vi "Send.vi"(8 "error in":errorcluster, 11 "Block Upload Transfer in":refnum<class "Block Upload Sub-Block Transfer.lvclass">) -> (0 "error out":errorcluster, 3 "Block Upload Transfer out":refnum<class "Block Upload Sub-Block Transfer.lvclass">)   [LabVIEW 2020, in "CANopen.lvlib" / "SDO Manager.lvlib" / "Block Upload Sub-Block Transfer.lvclass"]
doc: "SDO block upload initiate (phase II)"
uses:
  Block Upload Sub-Block Transfer.lvclass
  D:/git/CANopen-LabVIEW/source/SDO/SDO Manager/SDO Transfer/SDO Transfer.lvclass
  SDO Transfer/SDO Transfer.lvclass/SDO Transfer.ctl
  CANopen Message/CANopen Message.lvclass/CANopen Message.ctl
  HAL/Source/Interfaces/ICommunicate/ICommunicate.lvclass
  CANopen Message/CANopen Message.lvclass
  Typedefs/Function Code.ctl
  CANopen.lvlib
  SDO Transfer/SDO Transfer.lvclass
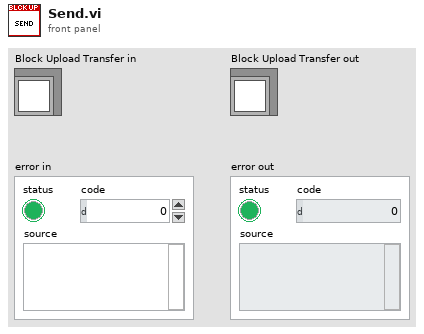
[diagram p1: front panel]
types:
  T1 = typedef "CANopen.lvlib/Function Code.ctl" = u8
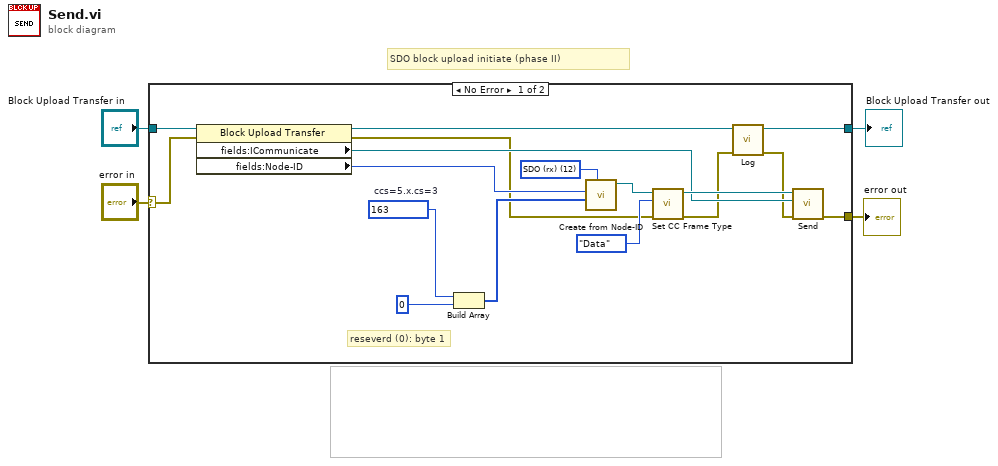
[diagram p0: block diagram]
diagram:
  # "SDO block upload initiate (phase II)"
  n1 = case shown="No Error" "error in" {
    selector: "error in" -> [w21 w22]
    tunnel: "Block Upload Transfer in" -> [w20 w23]
    tunnel: [w10 w23] -> w3
    tunnel: [w9 w22] -> w2
    frame No Error {
      w16 = T1 12 items=["NMT"=0, "EMCY/SYNC"=1, "TIME"=2, "PDO1 (tx)"=3, "PDO1 (rx)"=4, "PDO2 (tx)"=5, "PDO2 (rx)"=6, "PDO3 (tx)"=7, "PDO3 (rx)"=8, "PDO4 (tx)"=9, "PDO4 (rx)"=10, "SDO (tx)"=11, "SDO (rx)"=12, "NMT error control"=14] ("Function Code")
      w18 = u8 163  # ccs=5.x.cs=3
      # "reseverd (0): byte 1"
      n2 = property class="Block Upload Transfer"(reference=w20, error in=w21) -> (reference out=w11:refnum<class "Block Upload Sub-Block Transfer.lvclass">, error out=w8:errorcluster, "fields:ICommunicate"=w12:refnum<class "ICommunicate.lvclass">, "fields:Node-ID"=w19:u8)
      n3 = Build Array(w18, u8 0) -> (w17:u8[])
      n4 = call "Create from Node-ID.vi"("Function Code"=w16, "Data"=w17, "Node-ID"=w19) -> ("CANopen Message"=w15:refnum<class "CANopen Message.lvclass">)  [unwired: 8 in]
      n5 = call "Set CC Frame Type.vi"("error in"=w8, "CC Frame Type"=enum8{"Data", "Remote", "Error", "Overload"}."Data", "CANopen Message in"=w15) -> ("error out"=w7:errorcluster, "CANopen Message out"=w14:refnum<class "CANopen Message.lvclass">)  [unwired: 7 in]
      n6 = call "Log.vi"("error in"=w7, "SDO Transfer in"=w11) -> ("error out"=w6:errorcluster, "SDO Transfer out"=w10:refnum<class "Block Upload Sub-Block Transfer.lvclass">)  [unwired: 8 in]
      n7 = call "Send.vi"("error in"=w6, "ICommunicate"=w12, "CANopen Message in"=w14) -> ("error out"=w9:errorcluster)  [unwired: 7 in, 1 out]
    }
    frame Error {
    }
  }
  "Block Upload Transfer out" <- w3
  "error out" <- w2
